vi "VoltageCurrent.vi"(7 "Self-Calibrate at the beginning?":bool, 8 "Range (Volts)":dbl=10.0 format="%.2p", 9 "Resolution in Digits":T1=5.5 items=["3 1/2"=3.5, "4 1/2"=4.5, "5 1/2"=5.5, "6 1/2"=6.5, "7 1/2"=7.5], 10 "Function":T2, 11 "Instrument Descriptor":refnum<k15>) -> (0 "error out":errorcluster, 2 "Measurement (Volts)":dbl format="%_7p", 3 "instrument handle out":refnum<k15>, 5 "Over Range?":bool)   [LabVIEW 2019]
uses:
  <instrlib>/niDMM/nidmm.llb/niDMM Function.ctl
  <instrlib>/niDMM/nidmm.llb/niDMM Resolution in Digits.ctl
  <instrlib>/niDMM/nidmm.llb/niDMM Configure Measurement Digits.vi
panel:
  out "Waveform Chart":dbl(graph)
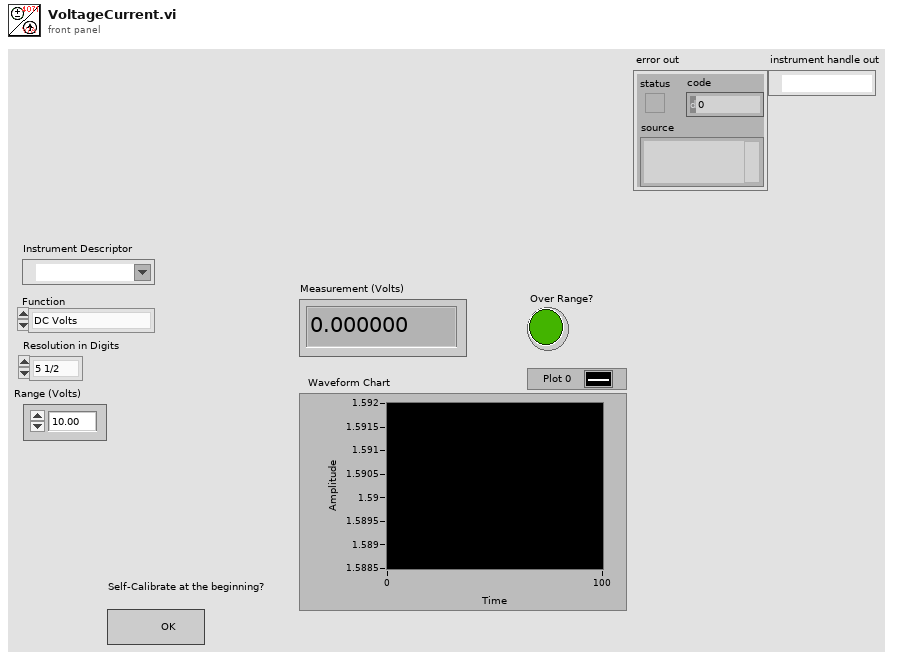
[diagram p1: front panel]
types:
  T1 = typedef "niDMM Resolution in Digits.ctl" = dbl
  T2 = typedef "niDMM Function.ctl" = enum16{"DC Volts", "AC Volts", "DC Current", "AC Current", "2-wire Resistance", "4-wire Resistance", "Diode", "Frequency", "Period", "AC Volts DC Coupled", "Capacitance", "Inductance", "Temperature"}
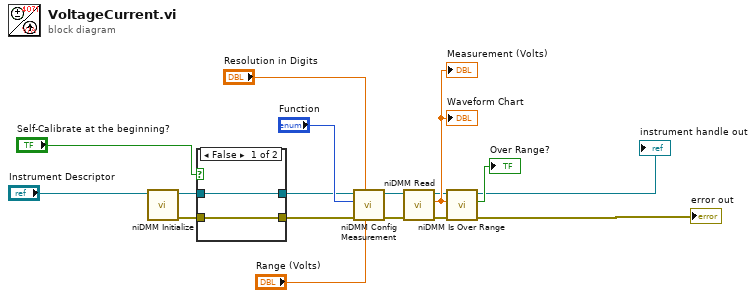
[diagram p0: block diagram]
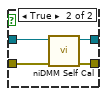
[diagram p2: hidden frame]
diagram:
  n1 = call <instrlib>:"niDMM Initialize.vi"("Instrument Descriptor"="Instrument Descriptor") -> ("error out"=w15:errorcluster, "instrument handle out"=w16:refnum<k15>)  [unwired: 9 in]
  n2 = case shown="False" "Self-Calibrate at the beginning?" {
    tunnel: w16 -> [w19 w23]
    tunnel: w15 -> [w18 w22]
    tunnel: [w18 w21] -> w4
    tunnel: [w19 w20] -> w3
    frame False {
    }
    frame True {
      n3 = call <instrlib>:"niDMM Self Cal.vi"("error in (no error)"=w22, "instrument handle"=w23) -> ("error out"=w21:errorcluster, "instrument handle out"=w20:refnum<k15>)  [unwired: 8 in]
    }
  }
  n4 = call-poly <instrlib>:"niDMM Config Measurement.vi"("Range"="Range (Volts)", "Resolution in Digits"="Resolution in Digits", "error in (no error)"=w4, "Function"="Function", "instrument handle"=w3) -> ("error out"=w8:errorcluster, "instrument handle out"=w7:refnum<k15>)  [unwired: 5 in]
  n5 = call <instrlib>:"niDMM Read.vi"("error in (no error)"=w8, "instrument handle"=w7) -> ("error out"=w10:errorcluster, "Measurement"=w12:dbl, "instrument handle out"=w9:refnum<k15>)  [unwired: 7 in]
  "Measurement (Volts)" <- w12
  "Waveform Chart" <- w12
  n6 = call <instrlib>:"niDMM Is Over Range.vi"("error in (no error)"=w10, "Measurement"=w12, "instrument handle"=w9) -> ("error out"=→"error out":errorcluster, "Over Range?"=→"Over Range?":bool, "instrument handle out"=→"instrument handle out":refnum<k15>)  [unwired: 6 in]
